vi "字符串转数字.vi"(8 "error in (no error)":errorcluster caption="错误输入（无错误）", 11 "字符串":string) -> (0 "error out":errorcluster caption="错误输出", 2 "数值":dbl, 3 "ID":i32)   [LabVIEW 2020]
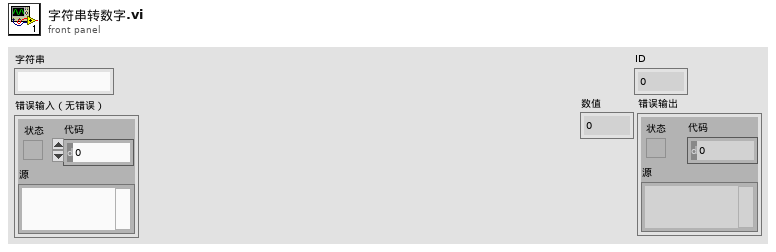
[diagram p1: front panel]
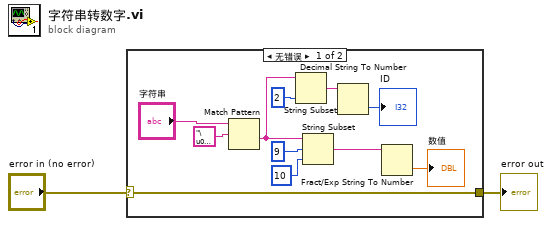
[diagram p0: block diagram]
diagram:
  n1 = case shown="无错误" "error in (no error)" {
    selector: "error in (no error)" -> [w3 w14]
    tunnel: [w3 w14] -> w1
    frame No Error {
      n2 = Match Pattern(string="字符串", regular expression="\u0002" ("正则表达式")) -> (after substring=w9:string)  [unwired: 1 in, 3 out]
      n3 = String Subset(string=w9, length (rest)=2 ("长度（剩余）")) -> (substring=w5:string)  [unwired: 1 in]
      n4 = String Subset(string=w9, offset (0)=9 ("偏移量(0)"), length (rest)=10 ("长度（剩余）")) -> (substring=w8:string)
      n5 = Decimal String To Number(string=w5) -> (number=→"ID":i32)  [unwired: 2 in, 1 out]
      n6 = Fract/Exp String To Number(string=w8) -> (number=→"数值":dbl)  [unwired: 3 in, 1 out]
    }
    frame Error {
    }
  }
  "error out" <- w1
